vi "Channels Array to Scan List.vi"(7 "GEt All":bool, 10 "Proc Num":i32=2, 11 "Channel-Grids":u16[][](array[ring])=[[1, 0, 0], [2, 0, 0], [3, 0, 0], [4, 0, 0], [5, 0, 0]] items=["NA", "1", "2", "3", "4", "5", "6", "7", "8", "9", "10", "11", "12", "13", "14", "15", "16", "17", "18", "19", "20"]) -> (2 "Channels":i32[](array[numeric]), 3 "Scan List":string)   [LabVIEW 2020]
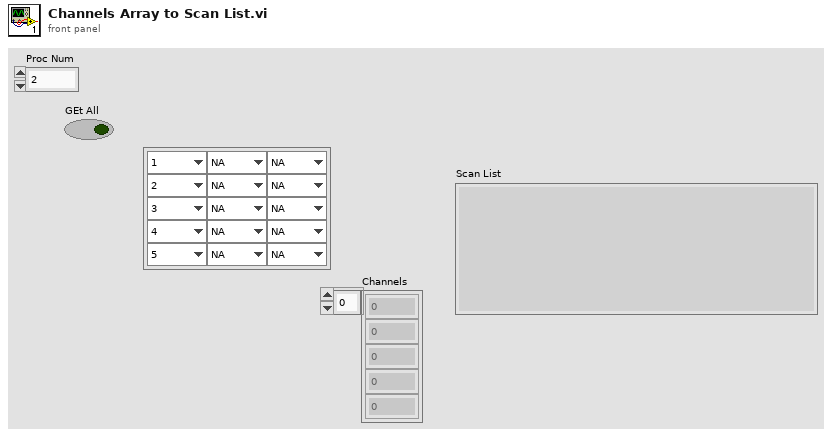
[diagram p1: front panel]
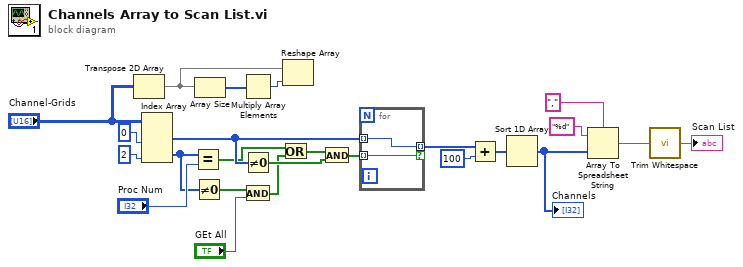
[diagram p0: block diagram]
diagram:
  n1 = Transpose 2D Array(2D array="Channel-Grids") -> (transposed array=w23:u16[][])
  n2 = Index Array(array="Channel-Grids", index (col) #1=0 ("disabled index (col)"), index (col) #2=2 ("index (col)")) -> (element #1=w10:u16[], element #2=w3:u16[])  [unwired: 2 in]
  n3 = Equal?(x=w3, y="Proc Num") -> (x = y?=w6:bool[])
  n4 = Not Equal To 0?(x=w3) -> (x != 0?=w1:bool[])
  n5 = Array Size(array=w23) -> (size(s)=w24:i32[])
  n6 = Multiply Array Elements(1:w24) -> (0:w22:i32)
  n7 = Not Equal To 0?(x=w10) -> (x != 0?=w18:bool[])
  n8 = And(x=w1, y="GEt All") -> (x .and. y?=w2:bool[])
  n9 = Or(x=w6, y=w2) -> (x .or. y?=w5:bool[])
  n10 = Reshape Array(w23, w22) -> ()  [unwired: 1 out]
  n11 = And(x=w5, y=w18) -> (x .and. y?=w8:bool[])
  n12 = for {
    tunnel: w8 -> [w25] mode=indexing
    tunnel: [w26] -> w17 mode=indexing if=w25
    tunnel: w10 -> [w26] mode=indexing
  }
  n13 = Add(x=w17, y=100) -> (x+y=w16:i32[])
  n14 = Sort 1D Array(array=w16) -> (sorted array=w15:i32[])
  "Channels" <- w15
  n15 = Array To Spreadsheet String(delimiter (Tab)=",", array=w15, 3:"%d" ("format string")) -> (spreadsheet string=w14:string)
  n16 = call <vilib>:"Trim Whitespace.vi"("string"=w14) -> ("trimmed string"=→"Scan List":string)  [unwired: 1 in]
